vi "Init.vi"(8 "error in (no error)":errorcluster, 10 "VISA name":refnum<visa-resource-name>="GPIB::5::INSTR", 11 "Low Level PSU In":refnum<class "Low Level PSU.lvclass">) -> (0 "error out":errorcluster, 3 "Low Level PSU Out":refnum<class "Low Level PSU.lvclass">)   [LabVIEW 2020, in "Low Level PSU.lvlib" / "Low Level PSU.lvclass"]
uses:
  Low Level PSU.lvclass
  Low Level PSU.lvclass/Low Level PSU.ctl
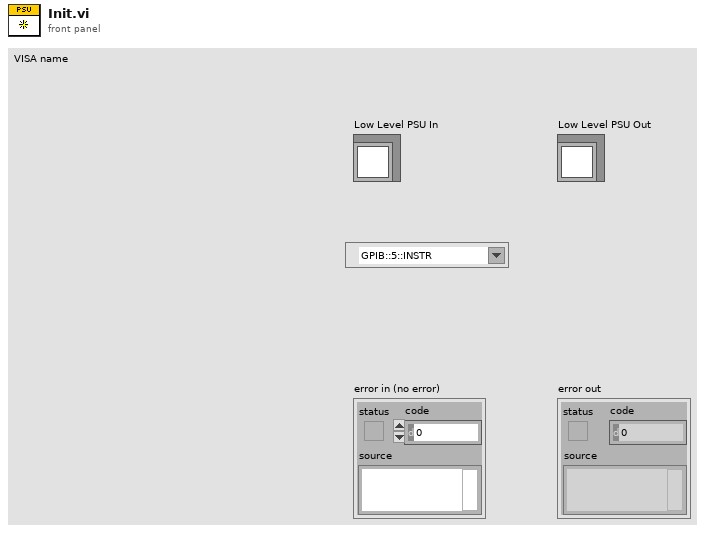
[diagram p1: front panel]
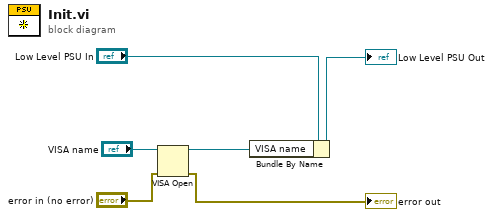
[diagram p0: block diagram]
diagram:
  n1 = VISA Open(error in (no error)="error in (no error)", VISA resource name="VISA name") -> (VISA resource name=w1:refnum<visa-resource-name>, error out=→"error out":errorcluster)  [unwired: 3 in]
  n2 = Bundle By Name(cluster="Low Level PSU In", "VISA name"=w1) -> (→"Low Level PSU Out":refnum<class "Low Level PSU.lvclass">)
